vi "Save.vi"(6 "current time":timestamp, 7 "base path":path, 8 "error in":errorcluster, 11 "Filename":string="<date>_exp<expno>_1.5to20") -> (0 "error out":errorcluster, 1 "#PicturesSavedOut":u32)   [LabVIEW 2016]
uses:
  controls/Enum.ctl
panel:
  in  "Nb of images recorded":dbl
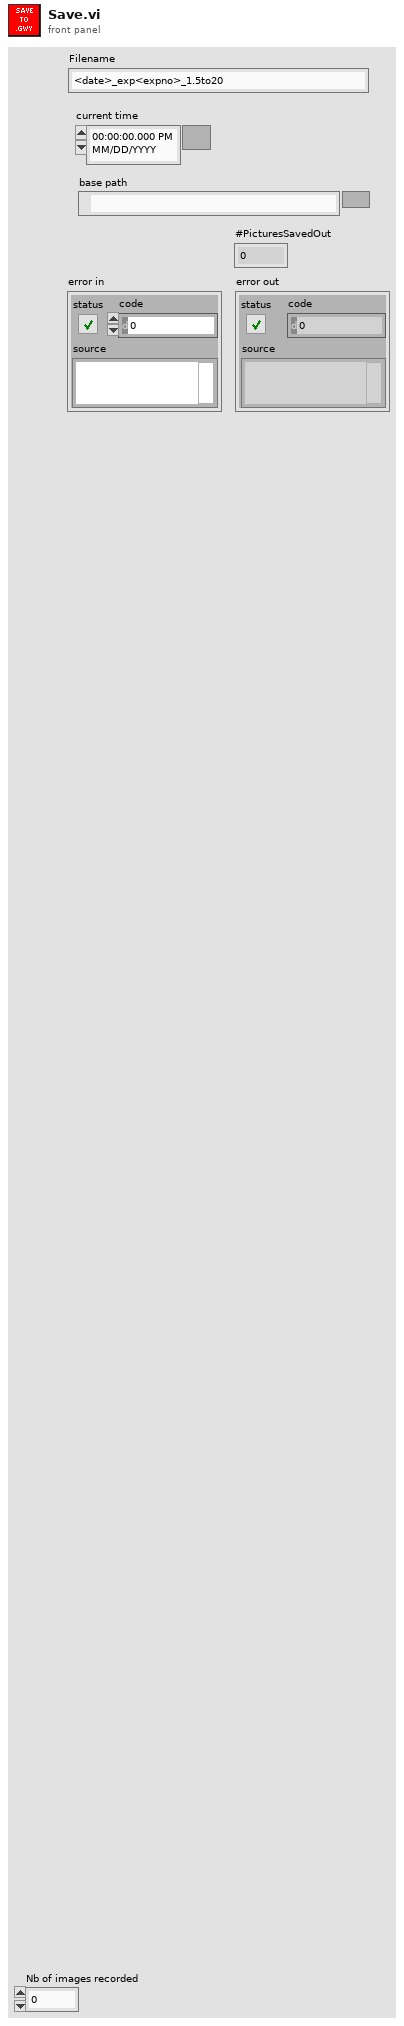
[diagram p1: front panel]
types:
  T1 = typedef "Enum.ctl" = enum16{"Init", "Read", "Write"}
  T2 = cluster{"Width":dbl, "Height":dbl, "X Offset":dbl, "Y Offset":dbl, "Angle":dbl, "Pixels/Line":u16, "Lines":u16, "Time/Line":dbl, "Scan Rate":dbl}
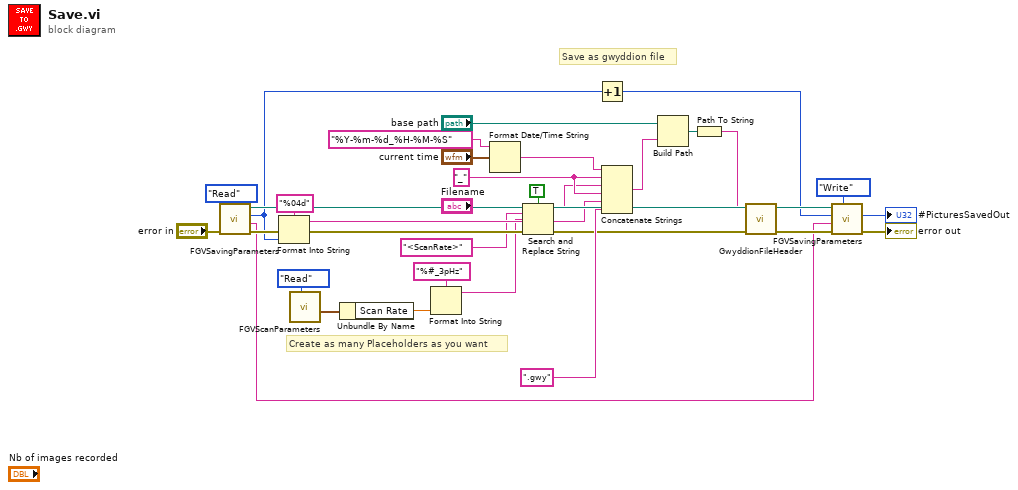
[diagram p0: block diagram]
diagram:
  w12 = "_" ("string")
  # "Create as many Placeholders as you want"
  # "Save as gwyddion file"
  n1 = call "FGVSavingParameters.vi"("Enum"=Enum."Read", "error in"="error in") -> ("error out"=w31:errorcluster, "filenameOut"=w16:string, "#PicturesSavedOut"=w17:u32, "pathOut"=w32:path)  [unwired: 6 in]
  n2 = Format Into String(format string="%04d", error in=w31, w17) -> (resulting string=w14:string, error out=w33:errorcluster)  [unwired: 1 in]
  n3 = call "FGVScanParameters.vi"("Enum"=Enum."Read") -> ("Scan Parameters Out"=w6:T2)  [unwired: 9 in, 1 out]
  n4 = Unbundle By Name(w6) -> ("Scan Rate"=w4:dbl)
  n5 = Format Into String(format string="%#_3pHz", w4) -> (resulting string=w3:string)  [unwired: 2 in, 1 out]
  n6 = Format Date/Time String(time format string (%c)="%Y-%m-%d_%H-%M-%S" ("format string"), seconds (now)="current time") -> (date/time string=w13:string)  [unwired: 1 in]
  n7 = Search and Replace String(case sensitive?=TRUE ("ignore case? (F)"), input string="Filename", search string="<ScanRate>" ("replace string (\"\")"), replace string=w3, error in=w33) -> (result string=w9:string, error out=w2:errorcluster)  [unwired: 3 in, 2 out]
  n8 = Increment(x=w17) -> (x+1=w19:u32)
  n9 = Concatenate Strings(w13, w12, w9, w12, w14, ".gwy" ("string")) -> (w23:string)
  n10 = Build Path(base path="base path", name or relative path=w23) -> (appended path=w18:path)
  n11 = Path To String(path=w18) -> (string=w30:string)
  n12 = call "GwyddionFileHeader.vi"("error in"=w2, "Filename"=w30) -> ("error out"=w27:errorcluster)  [unwired: 9 in]
  n13 = call "FGVSavingParameters.vi"("Enum"=Enum."Write", "error in"=w27, "filenameIn"=w16, "#PicturesSavedIn"=w19, "pathIn"=w32) -> ("error out"=→"error out":errorcluster, "#PicturesSavedOut"=→"#PicturesSavedOut":u32)  [unwired: 3 in, 2 out]
